vi "1WIRE_ROM_SEARCH_2.vi"(7 "1-Wire DIO Pin":refnum<k21>="ConnectorA/DIO15", 8 "Error In":errorcluster) -> (0 "Error Out":errorcluster, 2 "ROM Array":u64[](array[numeric]) format="%x")   [LabVIEW 2014]
uses:
  SearchROMvars.ctl
  <vilib>/rvi/Emulation/niFpgaGetClockAttributes.vi
  <vilib>/rvi/Emulation/niFpgaSctlEmulationGetInTimedLoop.vi
  <vilib>/rvi/Emulation/niFpgaEmulationReportErrorSimple.vi
  <vilib>/rvi/Emulation/niFpgaCriticalErrorInLSC.vi
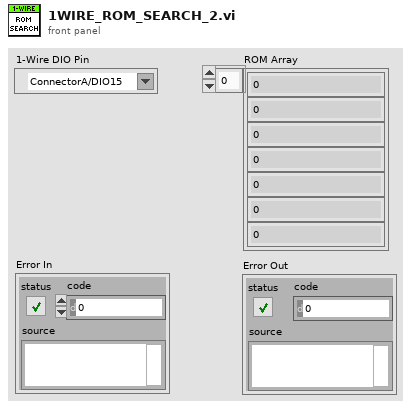
[diagram p1: front panel]
types:
  T1 = typedef "SearchROMvars.ctl" = cluster{"id_bit_number":i16, "comp_id_bit":bool, "id_bit":bool, "LastDeviceFlag":bool, "LastDiscrepancy":i16, "LastFamilyDiscrepancy":i16, "last_zero":i16, "ROM_NO":u64, "search_direction":bool}
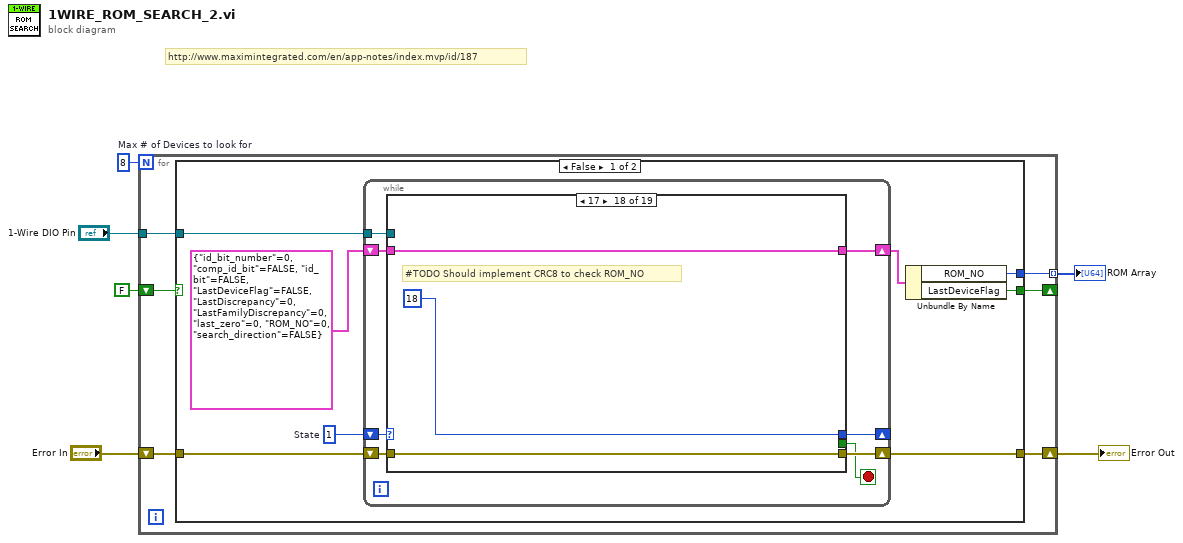
[diagram p0: block diagram]
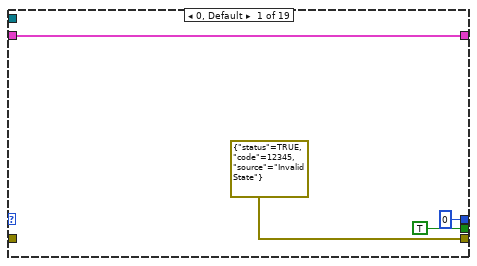
[diagram p2: hidden frame]
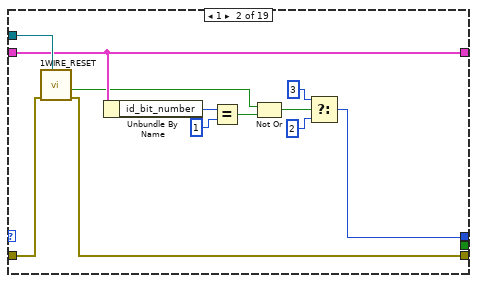
[diagram p3: hidden frame]
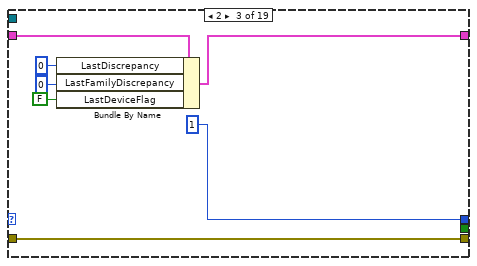
[diagram p4: hidden frame]
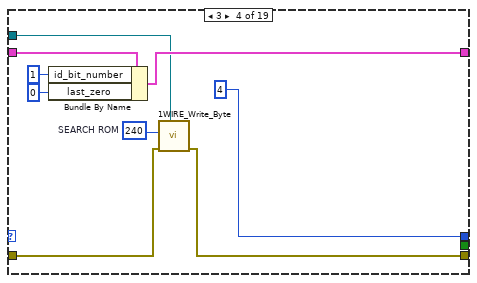
[diagram p5: hidden frame]
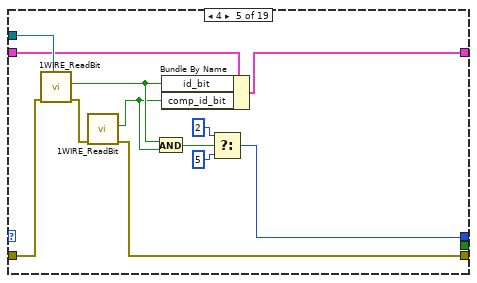
[diagram p6: hidden frame]
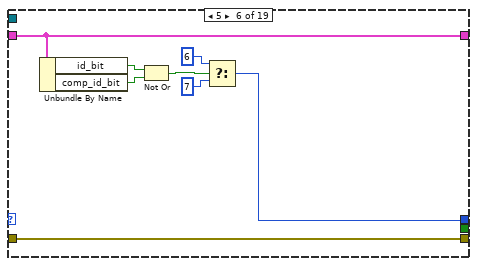
[diagram p7: hidden frame]
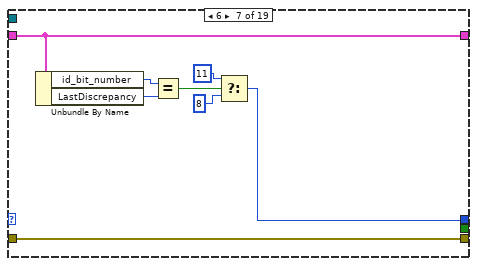
[diagram p8: hidden frame]
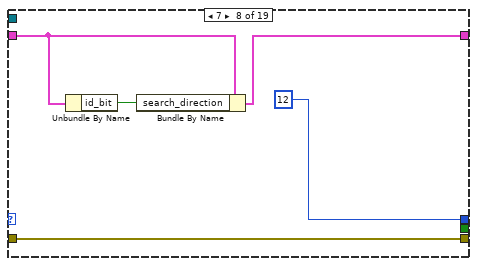
[diagram p9: hidden frame]
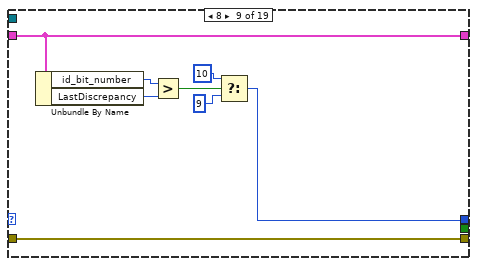
[diagram p10: hidden frame]
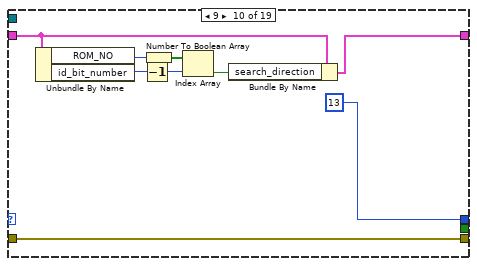
[diagram p11: hidden frame]
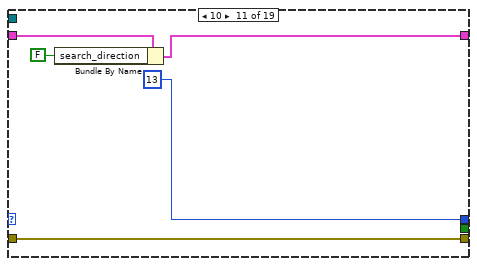
[diagram p12: hidden frame]
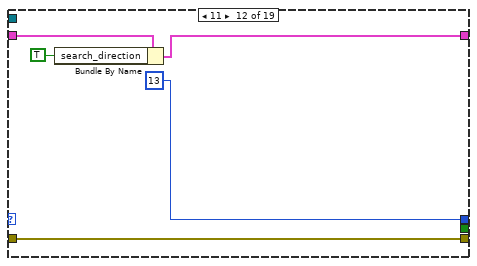
[diagram p13: hidden frame]
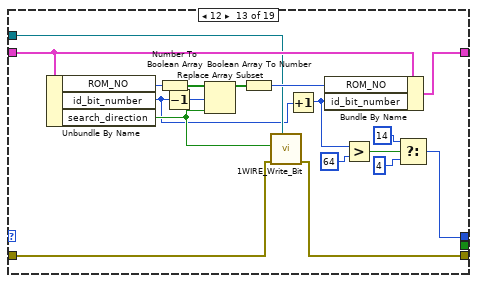
[diagram p14: hidden frame]
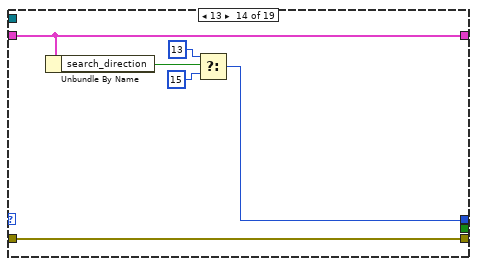
[diagram p15: hidden frame]
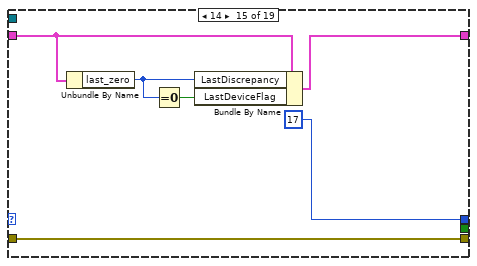
[diagram p16: hidden frame]
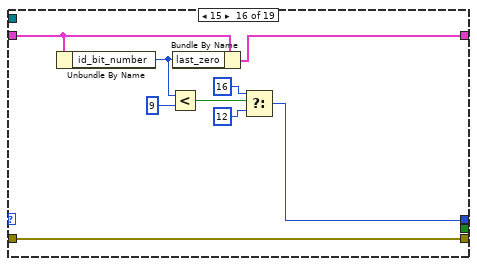
[diagram p17: hidden frame]
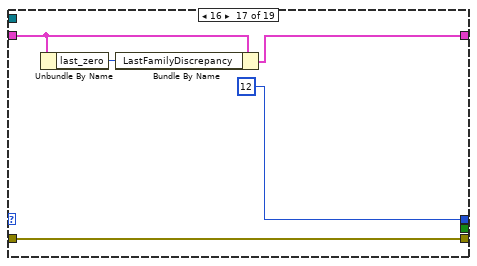
[diagram p18: hidden frame]
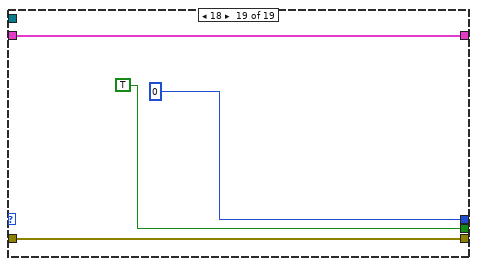
[diagram p19: hidden frame]
diagram:
  w2 = 8  # Max # of Devices to look for
  # "http://www.maximintegrated.com/en/app-notes/index.mvp/id/187"
  n1 = for {
    N: w2 -> [_]
    tunnel: "1-Wire DIO Pin" -> [w12]
    shift-right: [w10] -> w4
    shift-left: "Error In" -> [w11]
    tunnel: [w9] -> w3 mode=indexing
    shift-right: [w8] -> _
    shift-left: FALSE ("LastDeviceFlag") -> [w7]
    n2 = case shown="False" w7 {
      selector: w7 -> [_ w172]
      tunnel: w12 -> [w19 _]
      tunnel: w11 -> [w17 w173]
      tunnel: [w16 w173] -> w10
      tunnel: [w14 _] -> w9
      tunnel: [w13 w172] -> w8
      frame False {
        w20 = i16 1  # State
        n3 = while {
          shift-right: [w26] -> w15
          shift-left: T1 {"id_bit_number"=0, "comp_id_bit"=FALSE, "id_bit"=FALSE, "LastDeviceFlag"=FALSE, "LastDiscrepancy"=0, "LastFamilyDiscrepancy"=0, "last_zero"=0, "ROM_NO"=0, "search_direction"=FALSE} ("Cluster") -> [w25]
          shift-right: [w23] -> w16
          shift-left: w17 -> [w24]
          shift-right: [w22] -> _
          shift-left: w20 -> [w28]
          tunnel: w19 -> [w27]
          stop <- w21 stop-if-true
          n4 = case shown="17" w28 {
            tunnel: w27 -> [_ w44 _ w55 w71 _ _ _ _ _ _ _ w132 _ _ _ _ _ _]
            tunnel: [w32 w41 w49 w57 w67 w79 w87 w90 w100 w103 w113 w118 w135 w143 w149 w157 w162 w167 w171] -> w26
            tunnel: w25 -> [w32 w41 w50 w58 w68 w79 w87 w91 w100 w104 w114 w119 w136 w143 w148 w158 w163 w167 w171]
            tunnel: w24 -> [_ w43 w51 w54 w70 w80 w88 w93 w101 w110 w115 w120 w130 w144 w150 w159 w164 w166 w170]
            tunnel: [errorcluster {"status"=TRUE, "code"=12345, "source"="Invalid State"} ("Error In") w42 w51 w53 w69 w80 w88 w93 w101 w110 w115 w120 w129 w144 w150 w159 w164 w166 w170] -> w23
            tunnel: [i16 0 ("State") w33 i16 1 ("State") i16 4 ("y") w61 w73 w81 i16 12 ("State") w94 i16 13 ("State") i16 13 ("State") i16 13 ("State") w121 w139 i16 17 ("State") w151 i16 12 ("State") i16 18 ("State") i16 0 ("State")] -> w22
            tunnel: [TRUE _ _ _ _ _ _ _ _ _ _ _ _ _ _ _ _ _ TRUE] -> w21
            frame 0, Default {
            }
            frame 1 {
              n5 = call "1WIRE_RESET.vi"("1-Wire DIO Pin"=w44, "error in"=w43) -> ("error out"=w42:errorcluster, "0 = Device Present / 1=no"=w38:bool)  [unwired: 8 in]
              n6 = Unbundle By Name(w41) -> ("id_bit_number"=w40:i16)
              n7 = Equal?(x=w40, y=i16 1) -> (x = y?=w37:bool)
              n8 = Not Or(1:w37, 2:w38) -> (0:w36:bool)
              n9 = Select(t=i16 3 ("y"), s=w36, f=i16 2 ("y")) -> (s? t:f=w33:i16)
            }
            frame 2 {
              n10 = Bundle By Name(cluster=w50, "LastDiscrepancy"=i16 0, "LastFamilyDiscrepancy"=i16 0, "LastDeviceFlag"=FALSE) -> (w49:T1)
            }
            frame 3 {
              w56 = u8 240  # SEARCH ROM
              n11 = Bundle By Name(cluster=w58, "id_bit_number"=i16 1, "last_zero"=i16 0) -> (w57:T1)
              n12 = call "1WIRE_Write_Byte.vi"("1-Wire DIO Pin"=w55, "error in"=w54, "Tx data"=w56) -> ("error out"=w53:errorcluster)  [unwired: 7 in, 1 out]
            }
            frame 4 {
              n13 = call "1WIRE_ReadBit.vi"("1-Wire DIO Pin"=w71, "error in"=w70) -> ("error out"=w72:errorcluster, "Bit Read"=w66:bool)  [unwired: 8 in]
              n14 = call "1WIRE_ReadBit.vi"("error in"=w72) -> ("error out"=w69:errorcluster, "Bit Read"=w65:bool)  [unwired: 9 in]
              n15 = And(x=w66, y=w65) -> (x .and. y?=w64:bool)
              n16 = Bundle By Name(cluster=w68, "id_bit"=w66, "comp_id_bit"=w65) -> (w67:T1)
              n17 = Select(t=i16 2 ("State"), s=w64, f=i16 5 ("State")) -> (s? t:f=w61:i16)
            }
            frame 5 {
              n18 = Unbundle By Name(w79) -> ("id_bit"=w77:bool, "comp_id_bit"=w78:bool)
              n19 = Not Or(1:w78, 2:w77) -> (0:w74:bool)
              n20 = Select(t=i16 6 ("State"), s=w74, f=i16 7 ("State")) -> (s? t:f=w73:i16)
            }
            frame 6 {
              n21 = Unbundle By Name(w87) -> ("id_bit_number"=w85:i16, "LastDiscrepancy"=w86:i16)
              n22 = Equal?(x=w85, y=w86) -> (x = y?=w82:bool)
              n23 = Select(t=i16 11 ("State"), s=w82, f=i16 8 ("State")) -> (s? t:f=w81:i16)
            }
            frame 7 {
              n24 = Unbundle By Name(w91) -> ("id_bit"=w92:bool)
              n25 = Bundle By Name(cluster=w91, "search_direction"=w92) -> (w90:T1)
            }
            frame 8 {
              n26 = Unbundle By Name(w100) -> ("id_bit_number"=w98:i16, "LastDiscrepancy"=w99:i16)
              n27 = Greater?(x=w98, y=w99) -> (0:w95:bool)
              n28 = Select(t=i16 10 ("State"), s=w95, f=i16 9 ("State")) -> (s? t:f=w94:i16)
            }
            frame 9 {
              n29 = Unbundle By Name(w104) -> ("ROM_NO"=w108:u64, "id_bit_number"=w107:i16)
              n30 = Decrement(x=w107) -> (x-1=w106:i16)
              n31 = Number To Boolean Array(number=w108) -> (Boolean array=w109:bool[])
              n32 = Index Array(array=w109, index=w106) -> (element=w105:bool)
              n33 = Bundle By Name(cluster=w104, "search_direction"=w105) -> (w103:T1)
            }
            frame 10 {
              n34 = Bundle By Name(cluster=w114, "search_direction"=FALSE) -> (w113:T1)
            }
            frame 11 {
              n35 = Bundle By Name(cluster=w119, "search_direction"=TRUE) -> (w118:T1)
            }
            frame 12 {
              n36 = Unbundle By Name(w136) -> ("ROM_NO"=w137:u64, "id_bit_number"=w123:i16, "search_direction"=w131:bool)
              n37 = Number To Boolean Array(number=w137) -> (Boolean array=w138:bool[])
              n38 = Decrement(x=w123) -> (x-1=w128:i16)
              n39 = Replace Array Subset(array=w138, new element=w131, index=w128) -> (w133:bool[])
              n40 = Boolean Array To Number(Boolean array=w133) -> (number=w134:u64)
              n41 = call "1WIRE_Write_Bit.vi"("1-Wire DIO Pin"=w132, "Error In"=w130, "Bit"=w131) -> ("Error Out"=w129:errorcluster)  [unwired: 8 in]
              n42 = Increment(x=w123) -> (x+1=w124:i16)
              n43 = Bundle By Name(cluster=w136, "ROM_NO"=w134, "id_bit_number"=w124) -> (w135:T1)
              n44 = Greater?(x=w124, y=i16 64) -> (0:w125:bool)
              n45 = Select(t=i16 14 ("State"), s=w125, f=i16 4 ("State")) -> (s? t:f=w121:i16)
            }
            frame 13 {
              n46 = Unbundle By Name(w143) -> ("search_direction"=w140:bool)
              n47 = Select(t=i16 13 ("State"), s=w140, f=i16 15 ("State")) -> (s? t:f=w139:i16)
            }
            frame 14 {
              n48 = Unbundle By Name(w148) -> ("last_zero"=w147:i16)
              n49 = Equal To 0?(x=w147) -> (x = 0?=w146:bool)
              n50 = Bundle By Name(cluster=w148, "LastDiscrepancy"=w147, "LastDeviceFlag"=w146) -> (w149:T1)
            }
            frame 15 {
              n51 = Unbundle By Name(w158) -> ("id_bit_number"=w156:i16)
              n52 = Less?(x=w156, y=i16 9) -> (x < y?=w152:bool)
              n53 = Bundle By Name(cluster=w158, "last_zero"=w156) -> (w157:T1)
              n54 = Select(t=i16 16 ("State"), s=w152, f=i16 12 ("State")) -> (s? t:f=w151:i16)
            }
            frame 16 {
              n55 = Unbundle By Name(w163) -> ("last_zero"=w161:i16)
              n56 = Bundle By Name(cluster=w163, "LastFamilyDiscrepancy"=w161) -> (w162:T1)
            }
            frame 17 {
              # "#TODO Should implement CRC8 to check ROM_NO"
            }
            frame 18 {
            }
          }
        }
        n57 = Unbundle By Name(w15) -> ("ROM_NO"=w14:u64, "LastDeviceFlag"=w13:bool)
      }
      frame True {
      }
    }
  }
  "Error Out" <- w4
  "ROM Array" <- w3
